vi "SETPORT.vi"(8 "error in (no error)":errorcluster, 9 "Valor":string, 10 "Port":dbl, 11 "NXP in":refnum<class "NXP.lvclass">) -> (0 "error out":errorcluster, 3 "NXP out":refnum<class "NXP.lvclass">)   [LabVIEW 2019, in "NXP.lvclass"]
uses:
  NXP.lvclass
  NXP.lvclass/NXP.ctl
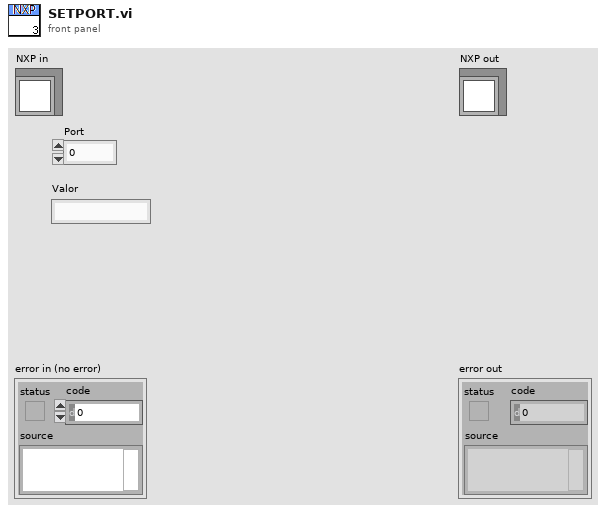
[diagram p1: front panel]
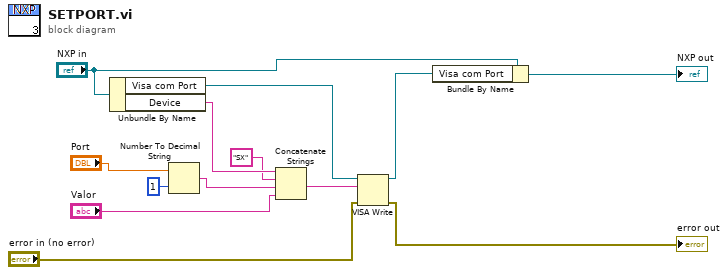
[diagram p0: block diagram]
diagram:
  n1 = Unbundle By Name("NXP in") -> ("Visa com Port"=w5:refnum<visa-resource-name>, "Device"=w9:string)
  n2 = Number To Decimal String(number="Port", width (-)=i16 1) -> (decimal integer string=w7:string)
  n3 = Concatenate Strings(w9, "SX" ("string"), w7, "Valor") -> (w4:string)
  n4 = VISA Write(VISA resource name=w5, write buffer=w4, error in (no error)="error in (no error)") -> (VISA resource name out=w1:refnum<visa-resource-name>, error out=→"error out":errorcluster)  [unwired: 1 out]
  n5 = Bundle By Name(cluster="NXP in", "Visa com Port"=w1) -> (→"NXP out":refnum<class "NXP.lvclass">)
